vi "TrajectoryCreateExecuteAbsolutePointInFront.vi"(8 "Init":bool, 11 "End Pose ENG":T1={"TRANSLATION"={"X"=0.0, "Y"=0.0}, "ROTATION"={"VALUE"=0.0, "COS"=1.0, "SIN"=0.0}} {"ROTATION"."SIN" format="%13.4f"; "ROTATION"."COS" format="%13.4f"; "ROTATION"."VALUE" format="%13.4f"; "TRANSLATION"."Y" format="%14.3f"; "TRANSLATION"."X" format="%14.3f"}) -> (0 "AtReference":bool, 2 "Done":bool, 3 "Chassis Velocity Target":T4 {"vOmega" format="%10.3f"; "vY" format="%10.3f"; "vX" format="%10.3f"})   [LabVIEW 2023]
uses:
  <vilib>/Rock Robotics/WPI/ThirdParty/JAS_Junk/TrajLib/TypeDef/CHASSIS_SPEEDS.ctl
  <vilib>/Rock Robotics/WPI/ThirdParty/JAS_Junk/TrajLib/TypeDef/POSE2D.ctl
  <vilib>/Rock Robotics/WPI/ThirdParty/JAS_Junk/TrajLib/TypeDef/TRANSLATION2D.ctl
  <vilib>/Rock Robotics/WPI/ThirdParty/JAS_Junk/TrajLib/TypeDef/ROTATION2D.ctl
  <vilib>/Rock Robotics/WPI/ThirdParty/JAS_Junk/TrajLib/VI/Util_GetTime_U32.vi
  <vilib>/Rock Robotics/WPI/ThirdParty/JAS_Junk/TrajLib/HolDrvCtrl_New.vi
  <vilib>/Rock Robotics/WPI/ThirdParty/JAS_Junk/TrajLib/HolDrvCtrl_PackPID.vi
  <vilib>/Rock Robotics/WPI/ThirdParty/JAS_Junk/TrajLib/HolDrvCtrl_SetTolerance.vi
  <vilib>/Rock Robotics/WPI/ThirdParty/JAS_Junk/TrajLib/HolDrvCtrl_SetEnabled.vi
  <vilib>/Rock Robotics/WPI/ThirdParty/JAS_Junk/TrajLib/HolDrvCtrl_Calculate_Trajectory.vi
  <vilib>/Rock Robotics/WPI/ThirdParty/JAS_Junk/TrajLib/HolDrvCtrl_AtReference.vi
  <vilib>/Rock Robotics/WPI/ThirdParty/JAS_Junk/TrajLib/Translation2d_GetXY.vi
  <vilib>/Rock Robotics/WPI/ThirdParty/JAS_Junk/TrajLib/Rotation2d_CreateXY.vi
  <vilib>/Rock Robotics/WPI/ThirdParty/JAS_Junk/TrajLib/Rotation2d_GetRadians.vi
  <vilib>/Rock Robotics/WPI/ThirdParty/JAS_Junk/TrajLib/PIDController_Pack_Tuning.vi
  <vilib>/Rock Robotics/WPI/ThirdParty/JAS_Junk/TrajLib/HolDrvCtrl_PackProfPID.vi
  <vilib>/Rock Robotics/WPI/ThirdParty/JAS_Junk/TrajLib/VI/HolDrvCtrl_PackControllers.vi
  <vilib>/Rock Robotics/WPI/ThirdParty/JAS_Junk/TrajLib/Pose2d_New.vi
  <vilib>/Rock Robotics/WPI/ThirdParty/JAS_Junk/TrajLib/ProfiledPIDController_EnableContInput.vi
  <vilib>/Rock Robotics/WPI/ThirdParty/JAS_Junk/TrajLib/Conv_Deg_Radians.vi
  <vilib>/Rock Robotics/WPI/ThirdParty/JAS_Junk/TrajLib/PIDController_NewPeriod.vi
  <vilib>/Rock Robotics/WPI/ThirdParty/JAS_Junk/TrajLib/PIDController_SetIntegratorRange.vi
  <vilib>/Rock Robotics/WPI/ThirdParty/JAS_Junk/TrajLib/PIDController_Reset.vi
  <vilib>/Rock Robotics/WPI/ThirdParty/JAS_Junk/TrajLib/HolDrvCtrl_Calculate.vi
  <vilib>/Rock Robotics/WPI/ThirdParty/JAS_Junk/TrajLib/Util_CalcDist.vi
  <vilib>/Rock Robotics/WPI/ThirdParty/JAS_Junk/TrajLib/ProfiledPIDController_NewPeriod.vi
  <vilib>/Rock Robotics/WPI/ThirdParty/JAS_Junk/TrajLib/ProfiledPIDController_SetIntegratorRange.vi
  <vilib>/Rock Robotics/WPI/ThirdParty/JAS_Junk/TrajLib/ProfiledPIDController_DisableContInput.vi
  <vilib>/Rock Robotics/WPI/ThirdParty/JAS_Junk/TrajLib/TrapProfConstraint_New.vi
  <vilib>/Rock Robotics/WPI/ThirdParty/JAS_Junk/TrajLib/Rotation2d_CreateAngle.vi
  <vilib>/Rock Robotics/WPI/ThirdParty/JAS_Junk/TrajLib/PIDController_EnableContinousInput.vi
  <vilib>/Rock Robotics/SystemInterfaces/NetworkCommunication/NetComm_UsageReport_report.vi
  <vilib>/Rock Robotics/WPI/ThirdParty/JAS_Junk/TrajLib/Rotation2d_GetAngleCosSin.vi
  <vilib>/Rock Robotics/WPI/ThirdParty/JAS_Junk/TrajLib/Pose2d_RelativeTo.vi
  <vilib>/Rock Robotics/WPI/ThirdParty/JAS_Junk/TrajLib/Pose2d_getRotation.vi
  <vilib>/Rock Robotics/WPI/ThirdParty/JAS_Junk/TrajLib/Rotation2d_Minus.vi
  <vilib>/Rock Robotics/WPI/ThirdParty/JAS_Junk/TrajLib/ProfiledPIDController_Calculate_Meas_Goal.vi
  <vilib>/Rock Robotics/WPI/ThirdParty/JAS_Junk/TrajLib/PIDController_Calculate_SP_PV.vi
  <vilib>/Rock Robotics/WPI/ThirdParty/JAS_Junk/TrajLib/ProfiledPIDController_Reset_PosOnly.vi
  <vilib>/Rock Robotics/WPI/ThirdParty/JAS_Junk/TrajLib/ChassisSpeeds_FromFieldRelativeSpeeds.vi
  <vilib>/Rock Robotics/WPI/ThirdParty/JAS_Junk/TrajLib/TrapProfState_New.vi
  <vilib>/Rock Robotics/WPI/ThirdParty/JAS_Junk/TrajLib/PIDController_DisableContinousInput.vi
  <vilib>/Rock Robotics/WPI/ThirdParty/JAS_Junk/TrajLib/Transform2d_Create_PosePose.vi
  <vilib>/Rock Robotics/WPI/ThirdParty/JAS_Junk/TrajLib/Pose2d_New_TRRO.vi
  <vilib>/Rock Robotics/WPI/ThirdParty/JAS_Junk/TrajLib/Rotation2d_UnaryMinus.vi
  <vilib>/Rock Robotics/WPI/ThirdParty/JAS_Junk/TrajLib/Rotation2d_RotateBy.vi
  <vilib>/Rock Robotics/WPI/ThirdParty/JAS_Junk/TrajLib/ProfiledPIDController_SetGoal_PosOnly.vi
  <vilib>/Rock Robotics/WPI/ThirdParty/JAS_Junk/TrajLib/ProfiledPIDController_Calculate_Meas.vi
  <vilib>/Rock Robotics/WPI/ThirdParty/JAS_Junk/TrajLib/PIDController_SetSetpoint.vi
  <vilib>/Rock Robotics/WPI/ThirdParty/JAS_Junk/TrajLib/PIDController_Calculate_PV.vi
  <vilib>/Rock Robotics/WPI/ThirdParty/JAS_Junk/TrajLib/ProfiledPIDController_Reset.vi
  <vilib>/Rock Robotics/WPI/ThirdParty/JAS_Junk/TrajLib/Rotation2d_GetCos.vi
  <vilib>/Rock Robotics/WPI/ThirdParty/JAS_Junk/TrajLib/Rotation2d_GetSin.vi
  <vilib>/Rock Robotics/WPI/ThirdParty/JAS_Junk/TrajLib/Translation2d_RotateBy.vi
  <vilib>/Rock Robotics/WPI/ThirdParty/JAS_Junk/TrajLib/ProfiledPIDController_SetGoal.vi
  <vilib>/Rock Robotics/WPI/ThirdParty/JAS_Junk/TrajLib/TrapProfile_New.vi
  <vilib>/Rock Robotics/WPI/ThirdParty/JAS_Junk/TrajLib/ProfiledPIDController_GetPeriod.vi
  <vilib>/Rock Robotics/WPI/ThirdParty/JAS_Junk/TrajLib/TrapProfile_Calculate.vi
  <vilib>/Rock Robotics/WPI/ThirdParty/JAS_Junk/TrajLib/ControllerUtil_GetModulusError.vi
  <vilib>/Rock Robotics/WPI/ThirdParty/JAS_Junk/TrajLib/TrapProfile_ShouldFlipAcceleration.vi
  <vilib>/Rock Robotics/WPI/ThirdParty/JAS_Junk/TrajLib/TrapProfile_Direct.vi
  <vilib>/Rock Robotics/WPI/ThirdParty/JAS_Junk/TrajLib/PIDController_GetPeriod.vi
  <vilib>/Rock Robotics/WPI/ThirdParty/JAS_Junk/TrajLib/Globals/Util_LibraryGlobals.vi
  Vision/VisionGlobal.vi
  TrajectoryGlobals.vi
  <vilib>/Rock Robotics/SystemInterfaces/Utilities/FPGA_UtilitiesRead LocalTime.vi
  <vilib>/Rock Robotics/WPI/ThirdParty/JAS_Junk/TrajLib/VI/Util_GetTime_U64.vi
  Drive/DriveGlobal.vi
  <vilib>/Rock Robotics/WPI/ThirdParty/JAS_Junk/TrajLib/Trajectory_Library.lvlib
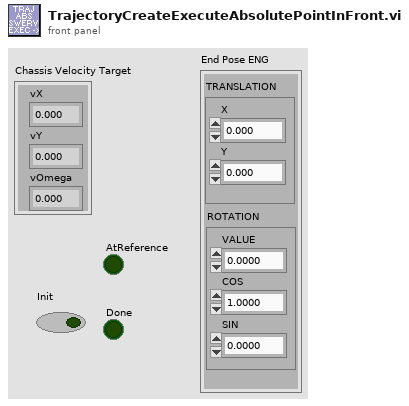
[diagram p1: front panel]
types:
  T1 = typedef "Trajectory_Library.lvlib/POSE2D.ctl" = cluster{"TRANSLATION":T2, "ROTATION":T3}
  T2 = typedef "Trajectory_Library.lvlib/TRANSLATION2D.ctl" = cluster{"X":dbl, "Y":dbl}
  T3 = typedef "Trajectory_Library.lvlib/ROTATION2D.ctl" = cluster{"VALUE":dbl, "COS":dbl, "SIN":dbl}
  T4 = typedef "Trajectory_Library.lvlib/CHASSIS_SPEEDS.ctl" = cluster{"vX":dbl, "vY":dbl, "vOmega":dbl}
  T5 = typedef "Trajectory_Library.lvlib/SWERVE_DRIVE_KINEMATICS.ctl" = cluster{"NumModules":i32, "InverseKinematics":T6, "ForwardKinematics":T6, "Modules":T2[], "PrevCoR":T2, "SavedModuleStates":T7[]}
  T6 = typedef "NI_Matrix.lvlib/RealMatrix.ctl" = dbl[][]
  T7 = typedef "Trajectory_Library.lvlib/SWERVE_DRIVE_MODULE_STATE.ctl" = cluster{"Speed":dbl, "Angle":T3}
  T8 = typedef "Trajectory_Library.lvlib/TRAJECTORY.ctl" = cluster{"TotalTImeSecs":dbl, "States":T9[]}
  T9 = typedef "Trajectory_Library.lvlib/TRAJ_STATE.ctl" = cluster{"TimeSeconds":dbl, "Velocity":dbl, "Acceleration":dbl, "POSE":T1, "Curvature":dbl}
  T10 = typedef "Trajectory_Library.lvlib/HOLONOMIC_PACK_TUNING.ctl" = cluster{"X PID Tuning":T11, "Y PID Tuning":T11, "thetaProfiledPID_CTRL":T12}
  T11 = typedef "Trajectory_Library.lvlib/PID_TUNING.ctl" = cluster{"Kp":dbl, "Ki":dbl, "Kd":dbl, "MaximumIntegral":dbl, "MinimumIntegral":dbl, "IntegralZone":dbl}
  T12 = typedef "Trajectory_Library.lvlib/PROFILED_PID_CONTROLLER.ctl" = cluster{"Controller":T13, "Goal":T14, "Setpoint":T14, "Constraint":T15}
  T13 = typedef "Trajectory_Library.lvlib/PID_CONTROLLER.ctl" = cluster{"Kp":dbl, "Ki":dbl, "Kd":dbl, "Period":dbl, "Max_Integral":dbl, "Min_Integral":dbl, "Max_Input":dbl, "Min_Input":dbl, "Continuous":bool, "PositionError":dbl, "VelocityError":dbl, "PrevError":dbl, "Total_Integral":dbl, "PositionTolerance":dbl, "VelocityTolerance":dbl, "SetPoint":dbl, "Kf":dbl, "Prev_Deriv":dbl, "Prev_Deriv 2":dbl, "DerivativeFilter":bool, "Min_Output":dbl, "Max_Output":dbl, "Prev_F_P":dbl, "Prev_F_P_2":dbl, "AntiWindupActive":bool, "Measurement":dbl, "IntegralZone":dbl}
  T14 = typedef "Trajectory_Library.lvlib/TRAPEZOID_PROFILE_STATE.ctl" = cluster{"Position":dbl, "Velocity":dbl}
  T15 = typedef "Trajectory_Library.lvlib/TRAPEZOID_PROFILE_CONSTRAINT.ctl" = cluster{"MaxVelocity":dbl, "MaxAcceleration":dbl}
  T16 = typedef "Trajectory_Library.lvlib/HOLONOMIC_DRV_CTRL.ctl" = cluster{"poseTolerance":T1, "poseError":T1, "Enabled":bool, "PID_xCtrl":T13, "PID_yCtrl":T13, "PROF_PID_thetaCtrl":T12, "RotationError":T3, "FirstRun":bool}
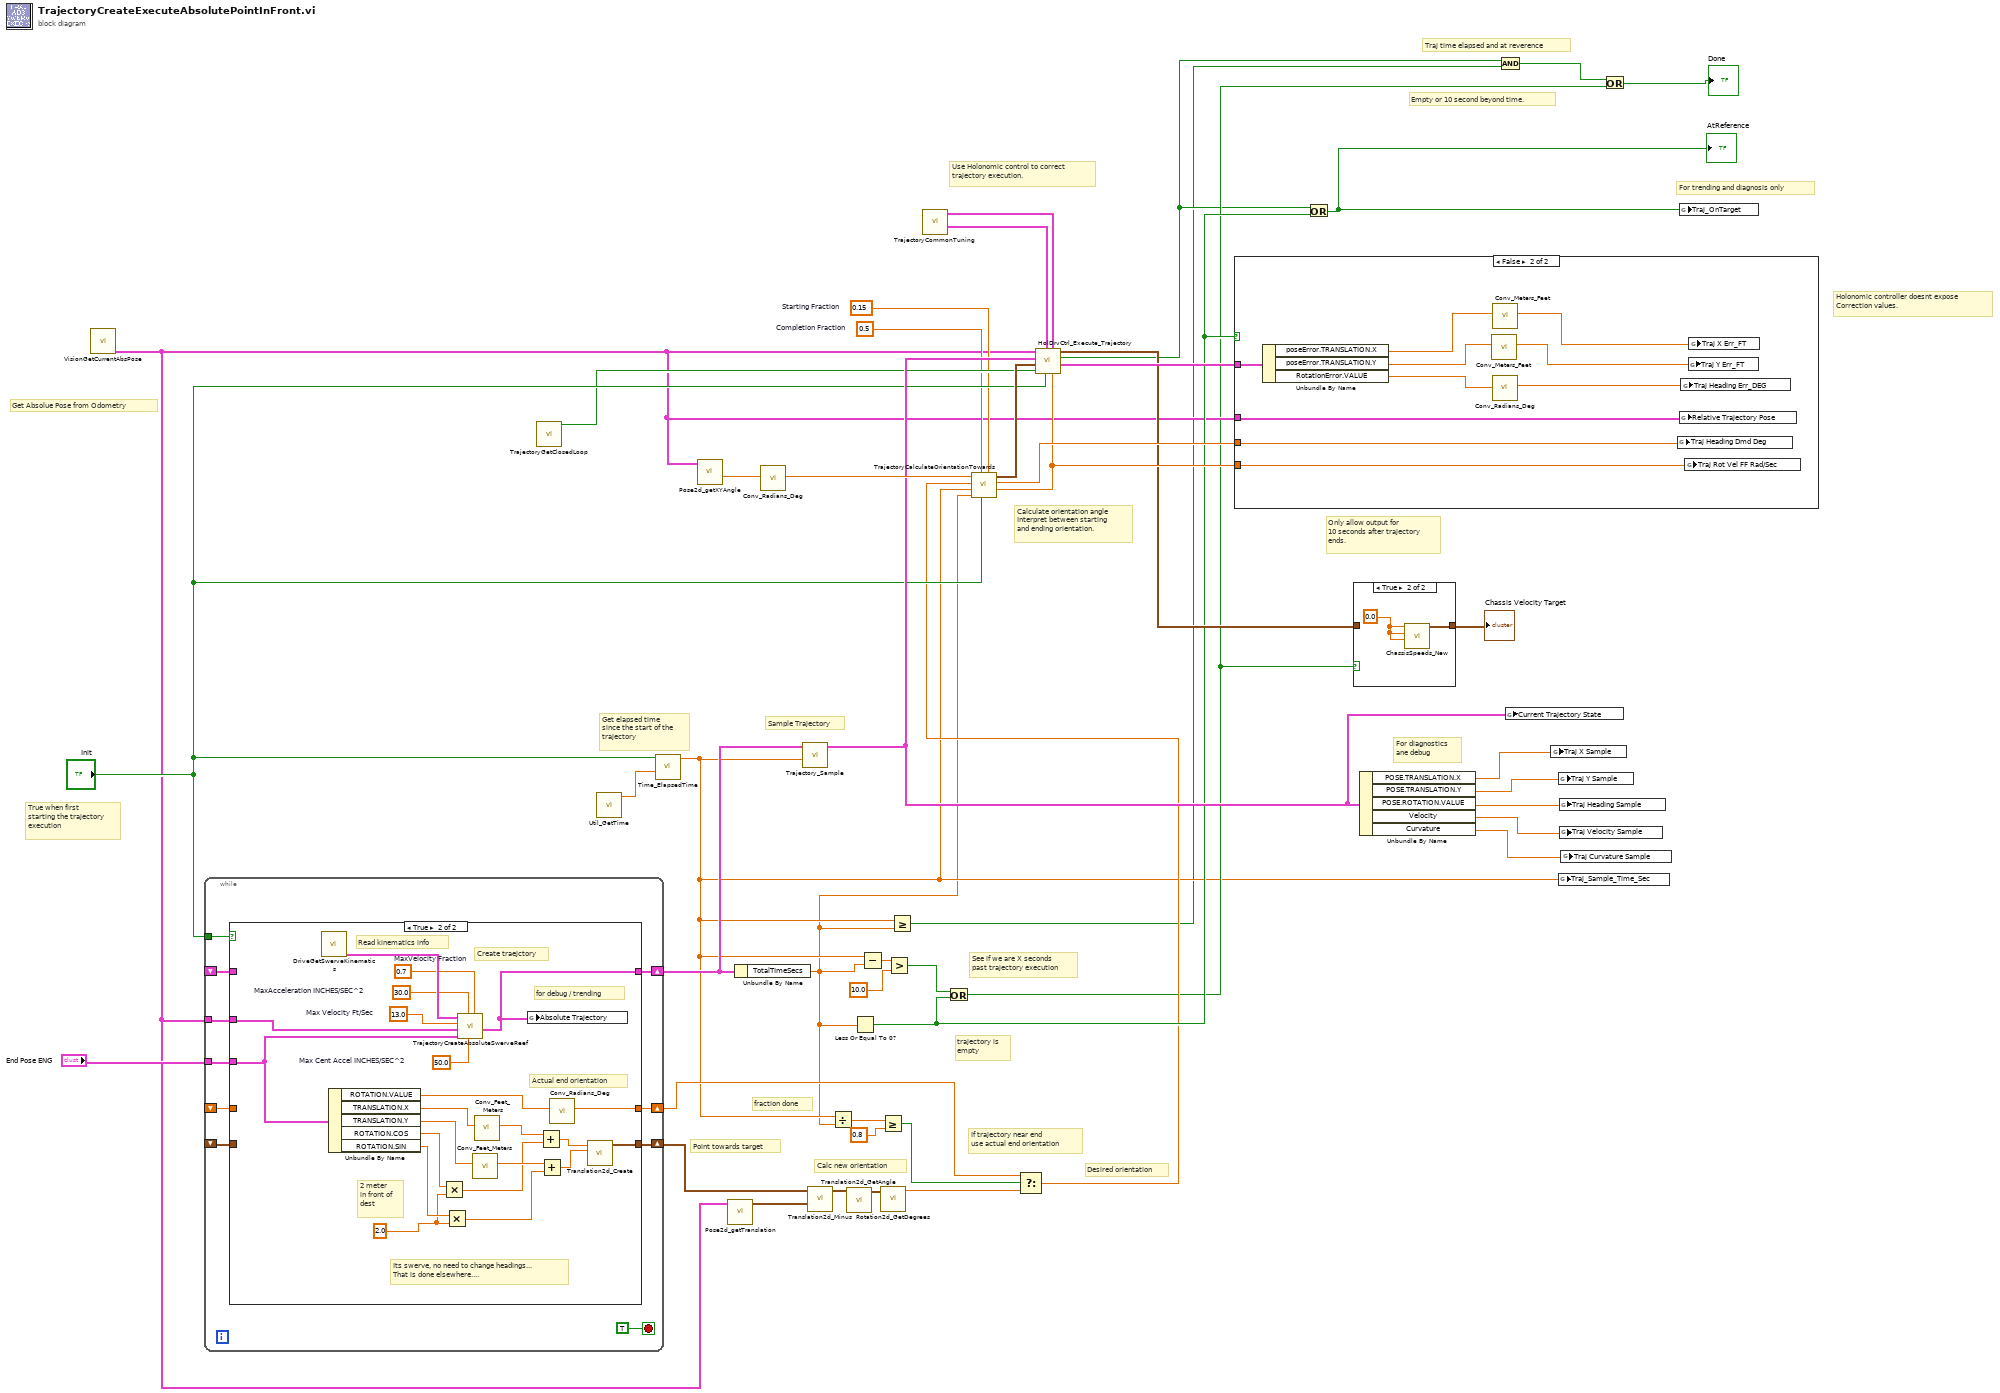
[diagram p0: block diagram]
diagram:
  w21 = 0.5  # Completion Fraction
  w22 = 0.15  # Starting Fraction
  # "Traj time elapsed and at reverence"
  # "Empty or 10 second beyond time."
  # "Desired orientation"
  # "fraction done"
  # "If trajectory near end\nuse actual end orientation"
  # "Calc new orientation"
  # "Point towards target"
  # "trajectory is \nempty"
  # "Calculate orientation angle\nInterpret between starting\nand ending orientation."
  # "True when first\nstarting the trajectory\nexecution"
  # "Get elapsed time\nsince the start of the\ntrajectory"
  # "Holonomic controller doesnt expose\nCorrection values."
  # "Use Holonomic control to correct\ntrajectory execution."
  # "For trending and diagnosis only"
  # "For diagnostics\nane debug"
  # "Get Absolue Pose from Odometry"
  # "Sample Trajectory"
  # "See if we are X seconds \npast trajectory execution"
  # "Only allow output for\n10 seconds after trajectory\nends."
  n1 = call "VisionGetCurrentAbsPose.vi"() -> ("Current ABS Pose"=w18:T1)  [unwired: 9 in]
  n2 = while {
    tunnel: "Init" -> [w55]
    tunnel: w18 -> [w54]
    shift-right: [w53] -> w33
    shift-left: _ -> [w52]
    shift-right: [w51] -> w11
    shift-left: _ -> [w50]
    tunnel: "End Pose ENG" -> [w49]
    shift-right: [w48] -> w17
    shift-left: _ -> [w47]
    stop <- TRUE stop-if-true
    n3 = case shown="True" w55 {
      tunnel: w54 -> [_ w78]
      tunnel: [w59 w79] -> w53
      tunnel: w52 -> [w59 _]
      tunnel: [w58 w81] -> w51
      tunnel: w50 -> [w58 _]
      tunnel: w49 -> [_ w64]
      tunnel: [w57 w65] -> w48
      tunnel: w47 -> [w57 _]
      frame False {
      }
      frame True {
        w60 = 0.7  # MaxVelocity Fraction
        w61 = 30.0  # MaxAcceleration INCHES/SEC^2
        w62 = 13.0  # Max Velocity Ft/Sec
        w63 = 50.0  # Max Cent Accel INCHES/SEC^2
        w70 = 2.0 ("y")
        # "Actual end orientation"
        # "2 meter\nin front of\ndest"
        # "for debug / trending"
        # "Read kinematics info"
        # "Its swerve, no need to change headings...\nThat is done elsewhere...."
        # "Create traejctory"
        n4 = call "DriveGetSwerveKinematics.vi"() -> ("SWERVE_DRIVE_KINEMATICS"=w77:T5)  [unwired: 11 in]
        n5 = Unbundle By Name(w64) -> ("ROTATION.VALUE"=w80:dbl, "TRANSLATION.X"=w76:dbl, "TRANSLATION.Y"=w75:dbl, "ROTATION.COS"=w72:dbl, "ROTATION.SIN"=w71:dbl)
        n6 = Multiply(x=w72, y=w70) -> (x*y=w69:dbl)
        n7 = Multiply(x=w71, y=w70) -> (x*y=w68:dbl)
        n8 = call "TrajectoryCreateAbsoluteSwerveReef.vi"("MaxVelocity Fraction"=w60, "Max Cent Accel INCHES/SEC^2"=w63, "MaxAcceleration INCHES/SEC^2"=w61, "End Pose  ENG"=w64, "Current Pose SI"=w78, "Max Velocity Ft/Sec"=w62, "SWERVE_DRIVE_KINEMATICS"=w77) -> ("Absolute Trajectory"=w79:T8)  [unwired: 2 in, 2 out]
        n9 = call <vilib>:"Conv_Feet_Meters.vi"("Feet"=w75) -> ("Meters"=w73:dbl)  [unwired: 10 in]
        n10 = call <vilib>:"Conv_Feet_Meters.vi"("Feet"=w76) -> ("Meters"=w74:dbl)  [unwired: 10 in]
        n11 = global write "TrajectoryGlobals.vi" "Absolute Trajectory"(w79) -> ()
        n12 = Add(x=w74, y=w69) -> (x+y=w67:dbl)
        n13 = Add(x=w73, y=w68) -> (x+y=w66:dbl)
        n14 = call <vilib>:"Conv_Radians_Deg.vi"("Radians"=w80) -> ("Degrees"=w81:dbl)  [unwired: 10 in]
        n15 = call <vilib>:"Translation2d_Create.vi"("Y"=w66, "X"=w67) -> ("TRANSLATION"=w65:T2)  [unwired: 9 in]
      }
    }
  }
  n16 = call "TrajectoryGetClosedLoop.vi"() -> ("AUTO_CLOSED_LOOP"=w23:bool)  [unwired: 11 in]
  n17 = call <vilib>:"Util_GetTime.vi"() -> ("FPGA_Time_Seconds"=w43:dbl)  [unwired: 9 in, 2 out]
  n18 = call <vilib>:"Time_ElapsedTime.vi"("PassthroughTime_SEC"=w43, "Reset"="Init") -> ("Elapsed Time Sec"=w3:dbl)  [unwired: 9 in]
  n19 = call <vilib>:"Pose2d_getXYAngle.vi"("in POSE"=w18) -> ("Angle"=w32:dbl)  [unwired: 8 in, 2 out]
  n20 = call <vilib>:"Pose2d_getTranslation.vi"("in POSE"=w18) -> ("outTRANSLATION"=w16:T2)  [unwired: 10 in]
  n21 = Unbundle By Name(w33) -> ("TotalTImeSecs"=w2:dbl)
  n22 = call <vilib>:"Conv_Radians_Deg.vi"("Radians"=w32) -> ("Degrees"=w31:dbl)  [unwired: 10 in]
  n23 = call <vilib>:"Trajectory_Sample.vi"("Time"=w3, "InputTRAJECTORY"=w33) -> ("OutputTRAJ_STATE"=w30:T9)  [unwired: 9 in]
  n24 = call <vilib>:"Translation2d_Minus.vi"("other Translation"=w16, "In Translation"=w17) -> ("Out Translation"=w20:T2)  [unwired: 9 in]
  n25 = Divide(x=w3, y=w2) -> (x/y=w13:dbl)
  n26 = call <vilib>:"Translation2d_GetAngle.vi"("In Translation"=w20) -> ("Angle_Rotation2d"=w19:T3)  [unwired: 10 in]
  n27 = Less Or Equal To 0?(x=w2) -> (x <= 0?=w25:bool)
  n28 = Subtract(x=w3, y=w2) -> (x-y=w46:dbl)
  n29 = Greater Or Equal?(x=w13, y=0.8) -> (x >= y?=w10:bool)
  n30 = call <vilib>:"Rotation2d_GetDegrees.vi"("in ROTATION"=w19) -> ("AngleDegrees"=w14:dbl)  [unwired: 10 in]
  n31 = Greater?(x=w46, y=10.0) -> (0:w27:bool)
  n32 = Greater Or Equal?(x=w3, y=w2) -> (x >= y?=w1:bool)
  n33 = call "TrajectoryCommonTuning.vi"() -> ("out POSe"=w8:T1, "HOLONOMIC_CTRL_PACK_TUNING"=w9:T10)  [unwired: 10 in]
  n34 = Or(x=w27, y=w25) -> (x .or. y?=w5:bool)
  n35 = Select(t=w11, s=w10, f=w14) -> (s? t:f=w15:dbl)
  n36 = call "TrajectoryCalculateOrientationTowards.vi"("Starting Fraction"=w22, "Init"="Init", "Completion Fraction"=w21, "Total Trajectory Time Sec"=w2, "Elapsed Traj Time Sec"=w3, "Current Orientation Demand DEG"=w15, "Starting Orientation  DEG"=w31) -> ("Rotational Velocity Rad Per Sec"=w34:dbl, "Orientation Demand Deg"=w37:dbl, "Orientation Demand"=w36:T3)  [unwired: 2 in]
  n37 = call <vilib>:"HolDrvCtrl_Execute_Trajectory.vi"("Rotational Velocity Feedforward \nRad/Sec"=w34, "HOLONOMIC_CTRL_PACK_TUNING"=w9, "Reset"="Init", "Tolerance"=w8, "Enable"=w23, "angleRef"=w36, "desiredTrajState"=w30, "currentPose"=w18) -> ("outHOLONOMIC_DRV_CTRL"=w35:T16, "AtReference"=w4:bool, "calcChassisSpeed"=w28:T4)  [unwired: 1 in]
  n38 = case shown="False" w25 {
    tunnel: w37 -> [_ w91]
    tunnel: w35 -> [_ w85]
    tunnel: w34 -> [_ w84]
    tunnel: w18 -> [_ w82]
    frame True {
    }
    frame False {
      n39 = Unbundle By Name(w85) -> ("poseError.TRANSLATION.X"=w89:dbl, "poseError.TRANSLATION.Y"=w88:dbl, "RotationError.VALUE"=w83:dbl)
      n40 = call <vilib>:"Conv_Meters_Feet.vi"("Meters"=w88) -> ("Feet"=w87:dbl)  [unwired: 10 in]
      n41 = call <vilib>:"Conv_Radians_Deg.vi"("Radians"=w83) -> ("Degrees"=w90:dbl)  [unwired: 10 in]
      n42 = call <vilib>:"Conv_Meters_Feet.vi"("Meters"=w89) -> ("Feet"=w86:dbl)  [unwired: 10 in]
      n43 = global write "TrajectoryGlobals.vi" "Traj Heading Dmd Deg"(w91) -> ()
      n44 = global write "TrajectoryGlobals.vi" "Relative Trajectory Pose"(w82) -> ()
      n45 = global write "TrajectoryGlobals.vi" "Traj Heading Err_DEG"(w90) -> ()
      n46 = global write "TrajectoryGlobals.vi" "Traj Rot Vel FF Rad/Sec"(w84) -> ()
      n47 = global write "TrajectoryGlobals.vi" "Traj Y Err_FT"(w87) -> ()
      n48 = global write "TrajectoryGlobals.vi" "Traj X Err_FT"(w86) -> ()
    }
  }
  n49 = Or(x=w4, y=w25) -> (x .or. y?=w26:bool)
  "AtReference" <- w26
  n50 = case shown="True" w5 {
    tunnel: w28 -> [w92 _]
    tunnel: [w92 w93] -> w44
    frame False {
    }
    frame True {
      w94 = 0.0 ("vX")
      n51 = call <vilib>:"ChassisSpeeds_New.vi"("vAngular"=w94, "vY"=w94, "vX"=w94) -> ("CHASSIS"=w93:T4)  [unwired: 8 in]
    }
  }
  "Chassis Velocity Target" <- w44
  n52 = Unbundle By Name(w30) -> ("POSE.TRANSLATION.X"=w42:dbl, "POSE.TRANSLATION.Y"=w41:dbl, "POSE.ROTATION.VALUE"=w40:dbl, "Velocity"=w39:dbl, "Curvature"=w38:dbl)
  n53 = And(x=w4, y=w1) -> (x .and. y?=w6:bool)
  n54 = global write "TrajectoryGlobals.vi" "Current Trajectory State"(w30) -> ()
  n55 = global write "TrajectoryGlobals.vi" "Traj X Sample"(w42) -> ()
  n56 = global write "TrajectoryGlobals.vi" "Traj Y Sample"(w41) -> ()
  n57 = global write "TrajectoryGlobals.vi" "Traj_Sample_Time_Sec"(w3) -> ()
  n58 = global write "TrajectoryGlobals.vi" "Traj Heading Sample"(w40) -> ()
  n59 = global write "TrajectoryGlobals.vi" "Traj Velocity Sample"(w39) -> ()
  n60 = global write "TrajectoryGlobals.vi" "Traj Curvature Sample"(w38) -> ()
  n61 = Or(x=w6, y=w5) -> (x .or. y?=→"Done":bool)
  n62 = global write "TrajectoryGlobals.vi" "Traj_OnTarget"(w26) -> ()
